vi "Real LU Factor.vi"(0 "A":T1) -> (1 "LU Info":cluster{"LU":dbl[][], "Pivot":i32[]} {"LU" format="%.3f"}, 2 "sign":i32, 3 "error":i32)   [LabVIEW 2018, in "NI_AALBase.lvlib"]
uses:
  NI_AALBase.lvlib
  RealMatrix.ctl
  <resource>/lvanlys.dll
  NI_Matrix.lvlib
panel:
  # "Real LU Factor"
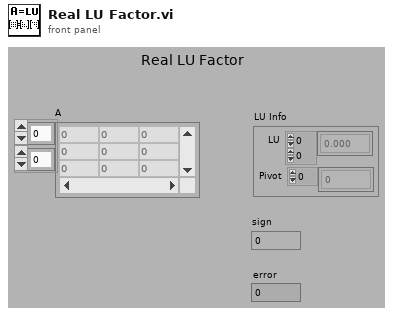
[diagram p1: front panel]
types:
  T1 = typedef "NI_Matrix.lvlib/RealMatrix.ctl" = dbl[][]
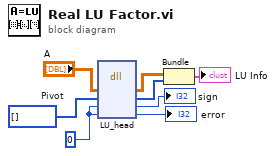
[diagram p0: block diagram]
diagram:
  w1 = 0 ("error")
  w6 = i32[] []  # Pivot
  n1 = dll-call lib="C:/Program Files (x86)/National Instruments/LabVIEW 2018/resource/lvanlys.*" fn="LU_head"("A"="A", "Pivot"=w6, "sign"=w1, "error"=w1) -> ("A"=w7:T1, "Pivot"=w5:i32[], "sign"=→"sign":i32, "error"=→"error":i32)  [unwired: 4 in, 2 out]
  n2 = Bundle("A"=w7, "Pivot"=w5) -> (→"LU Info":cluster{"A":T1, "Pivot":i32[]})  [unwired: 1 in]
